vi "PQerrorMessage.vi"(8 "error in (no error)":errorcluster, 11 "conn":u32) -> (0 "error out":errorcluster, 3 "PQerrorMessage":string, 5 "conn_out":u32)   [LabVIEW 2017, in "libpqlv.lvlib"]
doc: "Returns the error message most recently generated by an operation on the connection."
uses:
  libpqlv.lvlib
  lib/libpq.dll
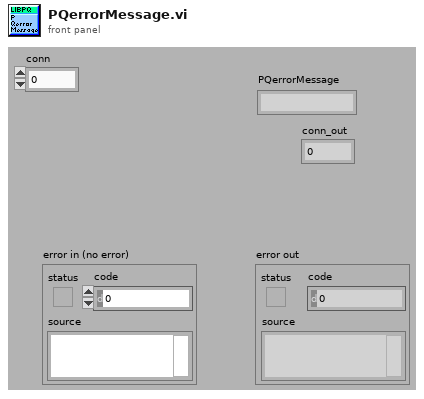
[diagram p1: front panel]
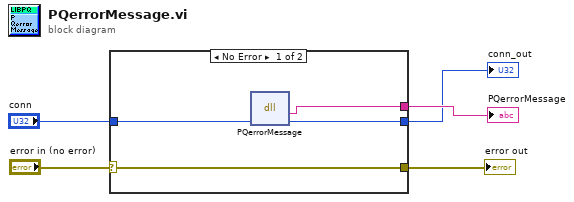
[diagram p0: block diagram]
diagram:
  n1 = case shown="No Error" "error in (no error)" {
    selector: "error in (no error)" -> [w9 w11]
    tunnel: [w9 w11] -> w4
    tunnel: [w8 _] -> w3
    tunnel: "conn" -> [w7 w10]
    tunnel: [w6 w10] -> w1
    frame No Error {
      n2 = dll-call lib="D:/Users/erics/Documents/active/DAQ/PostgreSQL2LabVIEW/libpqlv/lib/libpq.*" fn="PQerrorMessage"("conn"=w7) -> ("PQerrorMessage"=w8:string, "conn"=w6:u32)  [unwired: 3 in, 2 out]
    }
    frame Error {
    }
  }
  "PQerrorMessage" <- w3
  "error out" <- w4
  "conn_out" <- w1
